vi "UsrProfiles-Window-New User Name Entry.vi"(7 "Colour":u32(colorbox)=16777225, 8 "error in (no error)":errorcluster) -> (0 "error out":errorcluster, 1 "Cancelled (Left button pressed)":bool, 2 "New user name":string)   [LabVIEW 2013]
doc: "Use this template to create a dialog box with event handling."
uses:
  <vilib>/Utility/miscctls.llb/LVPointTypeDef.ctl
  Global Variables/General Globals.vi
panel:
  in  "User name":string caption="Enter new user name"
  in  "Cancel":bool
  in  "OK":bool
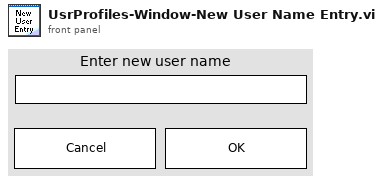
[diagram p1: front panel]
types:
  T1 = typedef "LVPointTypeDef.ctl" = cluster{"Horizontal":i16, "Vertical":i16}
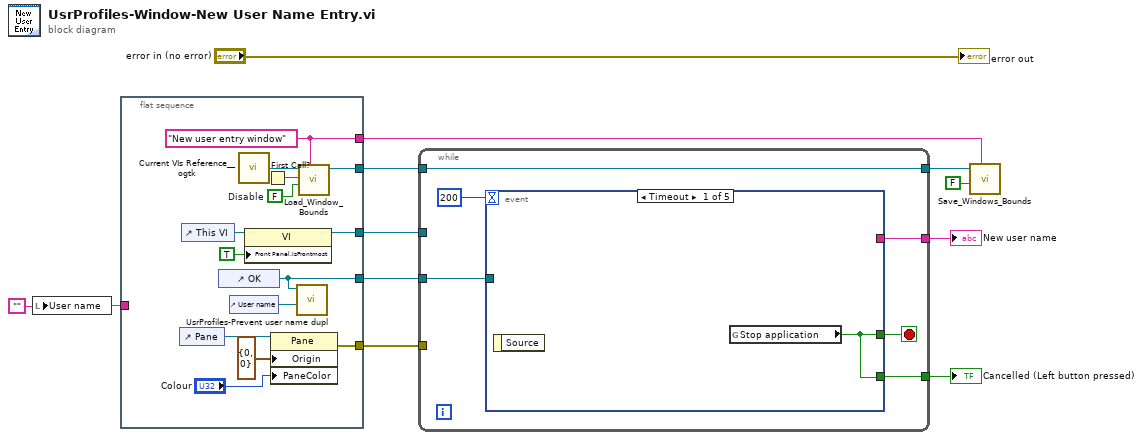
[diagram p0: block diagram]
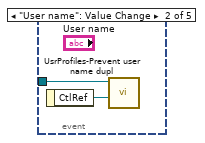
[diagram p2: hidden frame]
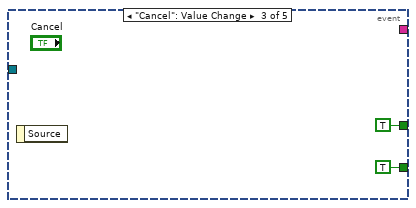
[diagram p3: hidden frame]
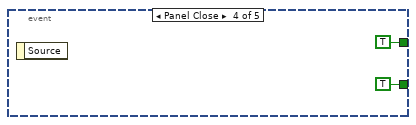
[diagram p4: hidden frame]
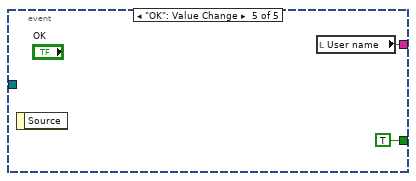
[diagram p5: hidden frame]
diagram:
  w1 = "" ("Name")
  n1 = local write "User name"(w1) -> ()
  n2 = flat-sequence {
    tunnel: [w23] -> w11
    tunnel: [w21] -> w10
    tunnel: [w16] -> w8
    tunnel: [w15] -> w6
    tunnel: [w13] -> w2
    tunnel: w1 -> [_]
    frame #0 {
      w17 = FALSE  # Disable
      w16 = "New user entry window" ("Window Name (i.e. Key)")
      n3 = control-ref of="Pane"() -> (w20:refnum<vi>)
      n4 = control-ref of="This VI"() -> (w24:refnum<vi>)
      n5 = control-ref of="OK"() -> (w13:refnum<vi>)
      n6 = control-ref of="User name"() -> (w12:refnum<vi>)
      n7 = call "Current VIs Reference__ogtk.vi"() -> ("Current VI's reference"=w19:refnum<vi>)  [unwired: 5 in]
      n8 = property on="Property Node" class="VI"(reference=w24, "Front Panel.IsFrontmost"=TRUE ("Front Panel Window:Is Frontmost")) -> (reference out=w23:refnum<vi>)  [unwired: 1 in, 1 out]
      n9 = First Call?() -> (First Call?: T/F=w18:bool)
      n10 = property class="Pane"(reference=w20, "Origin"=T1 {"Horizontal"=0, "Vertical"=0}, "PaneColor"="Colour") -> (error out=w21:errorcluster)  [unwired: 1 in, 1 out]
      n11 = call "UsrProfiles-Prevent user name dupl.vi"("User name ref"=w12, "OK button ref"=w13) -> ()  [unwired: 10 in]
      n12 = call "Load_Window_Bounds.vi"("Window Name (i.e. Key)"=w16, "Disable"=w17, "First Call"=w18, "Window VI's Ref"=w19) -> ("reference out"=w15:refnum<vi>)  [unwired: 4 in, 3 out]
    }
  }
  n13 = while {
    tunnel: w10 -> [_]
    tunnel: w11 -> [_]
    tunnel: [w29] -> w9
    tunnel: w6 -> [w28]
    tunnel: [w28] -> w5
    tunnel: [w26] -> w3
    tunnel: w2 -> [w27]
    stop <- w31 stop-if-true
    n14 = event shown="[0] Timeout" {
      selector: _ -> [_ _ _ _ _]
      dyn-events: _ -> [_ _ _ _ _]
      timeout: 200 -> [_ _ _ _ _]
      tunnel: [w32 _ TRUE ("Stop?") TRUE ("Stop?") TRUE ("Stop?")] -> w31
      tunnel: [w32 _ TRUE ("Stop subpanel") TRUE ("Stop subpanel") _] -> w29
      tunnel: w27 -> [_ w34 _ _ _]
      tunnel: [_ _ _ _ w39] -> w26
      event Timeout {
        n15 = event-data() -> ()  [unwired: 1 in, 1 out]
        n16 = global read "General Globals.vi" "Stop application"() -> (w32:bool)
      }
      event "User name": Value Change {
        n17 = event-data() -> ("CtlRef"=w33:refnum<vi>)  [unwired: 1 in]
        n18 = call "UsrProfiles-Prevent user name dupl.vi"("User name ref"=w33, "OK button ref"=w34) -> ()  [unwired: 10 in]
      }
      event "Cancel": Value Change {
        n19 = event-data() -> ()  [unwired: 1 in, 1 out]
      }
      event Panel Close {
        n20 = event-data() -> ()  [unwired: 1 in, 1 out]
      }
      event "OK": Value Change {
        n21 = event-data() -> ()  [unwired: 1 in, 1 out]
        n22 = local read "User name"() -> (w39:string)
      }
    }
  }
  "Cancelled (Left button pressed)" <- w9
  "New user name" <- w3
  n23 = call "Save_Windows_Bounds.vi"("Window Name (i.e. Key)"=w8, "Front Panel Window:Open"=FALSE, "Window VI's Ref"=w5) -> ()  [unwired: 8 in, 1 out]
  "error out" <- "error in (no error)"
